vi "Pause I2C Data.vi"(8 "error in (no error)":errorcluster, 11 "PauseResume Ref":refnum<vi>) -> (0 "error out":errorcluster, 2 "I2C Data":string[][](array[string]))   [LabVIEW 2025, in "I2C Bus Monitor UI.lvlib"]
uses:
  I2C Bus Monitor UI.lvlib
  Table Buffer - Dequeue.vi
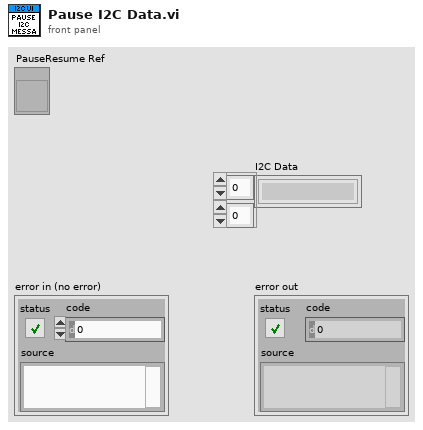
[diagram p1: front panel]
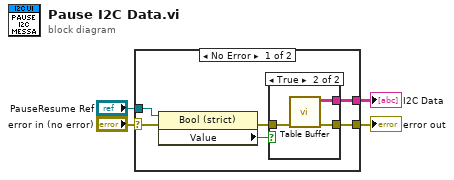
[diagram p0: block diagram]
diagram:
  n1 = case shown="No Error" "error in (no error)" {
    selector: "error in (no error)" -> [w9 w15]
    tunnel: [w10 w15] -> w4
    tunnel: "PauseResume Ref" -> [w7 _]
    tunnel: [w5 _] -> w1
    frame No Error {
      n2 = property class="Bool (strict)"(reference=w7, error in=w9) -> (error out=w8:errorcluster, "Value"=w6:bool)  [unwired: 1 out]
      n3 = case shown="True" w6 {
        tunnel: [w11 w14] -> w10
        tunnel: w8 -> [w11 w13]
        tunnel: [_ w12] -> w5
        frame False {
        }
        frame True {
          n4 = call-poly "Table Buffer.vi"("error in (no error)"=w13) -> ("error out"=w14:errorcluster, "Data"=w12:string[][])  [unwired: 9 in]
        }
      }
    }
    frame Error {
    }
  }
  "error out" <- w4
  "I2C Data" <- w1
